vi "Enable Events.vi"(8 "error in (no error)":errorcluster, 11 "Enclave in":refnum<class "Enclave.lvclass">) -> (0 "error out":errorcluster, 3 "Enclave out":refnum<class "Enclave.lvclass">)   [LabVIEW 2022 SP3, in "Enclave.lvlib" / "Enclave.lvclass"]
uses:
  Enclave.lvclass
  Enclave.lvclass/Enclave.ctl
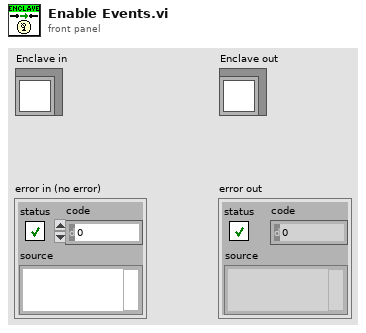
[diagram p1: front panel]
types:
  T1 = typedef "Enclave.lvlib/Writer Data.ctl" = cluster{"Queues":refnum<queue>[], "Lossy":bool, "Event":bool}
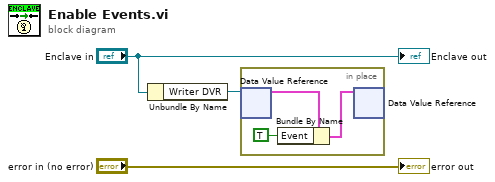
[diagram p0: block diagram]
diagram:
  n1 = Unbundle By Name("Enclave in") -> ("Writer DVR"=w1:refnum<data-value>)
  n2 = in-place {
    n3 = in-place-dvr #1(w1) -> (w6:T1)  [unwired: 1 out]
    n4 = Bundle By Name(cluster=w6, "Event"=TRUE) -> (w4:T1)
    n5 = in-place-dvr #1(w4) -> ()  [unwired: 2 out]
  }
  "error out" <- "error in (no error)"
  "Enclave out" <- "Enclave in"
